vi "两点至矩形（TB）.vi"(10 "point b":cluster{"x":i16, "y":i16} caption="点b", 11 "point a":cluster{"x":i16, "y":i16} caption="点a") -> (3 "RectTB":T1)   [LabVIEW 2011]
uses:
  RectTB.ctl
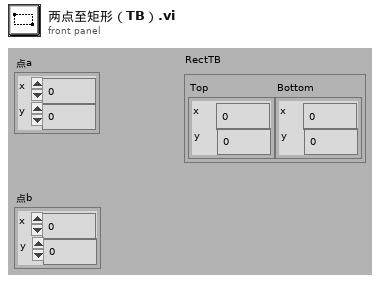
[diagram p1: front panel]
types:
  T1 = typedef "RectTB.ctl" = cluster{"Top":cluster{"x":i16, "y":i16}, "Bottom":cluster{"x":i16, "y":i16}}
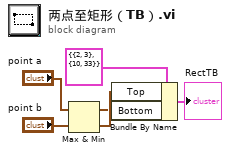
[diagram p0: block diagram]
diagram:
  n1 = Max & Min(x="point a", y="point b") -> (max(x,y)=w1:cluster{"x":i16, "y":i16}, min(x,y)=w2:cluster{"x":i16, "y":i16})
  n2 = Bundle By Name(cluster=T1 {"Top"={"x"=2, "y"=3}, "Bottom"={"x"=10, "y"=33}} ("RectTB"), "Top"=w2, "Bottom"=w1) -> (→"RectTB":T1)
